vi "Host Train PID.vi"() -> ()   [LabVIEW 2018]
doc: "This example demonstrates the Traditional MeanShift algorithm to track an object in the image."
uses:
  <vilib>/userdefined/High Color/IMAQdx.ctl
  <vilib>/vision/driver/NI_Vision_Acquisition_Software.lvlib
panel:
  out "Control Signal":dbl(graph)
  out "DECODED MESSAGE":string
  in  "?":T1="cam1"
  in  "Run":bool
  out "Theta":cluster{"Double":dbl, dbl}(graph)
  in  "Stop":bool
  out "Image":T2(plugin-control)
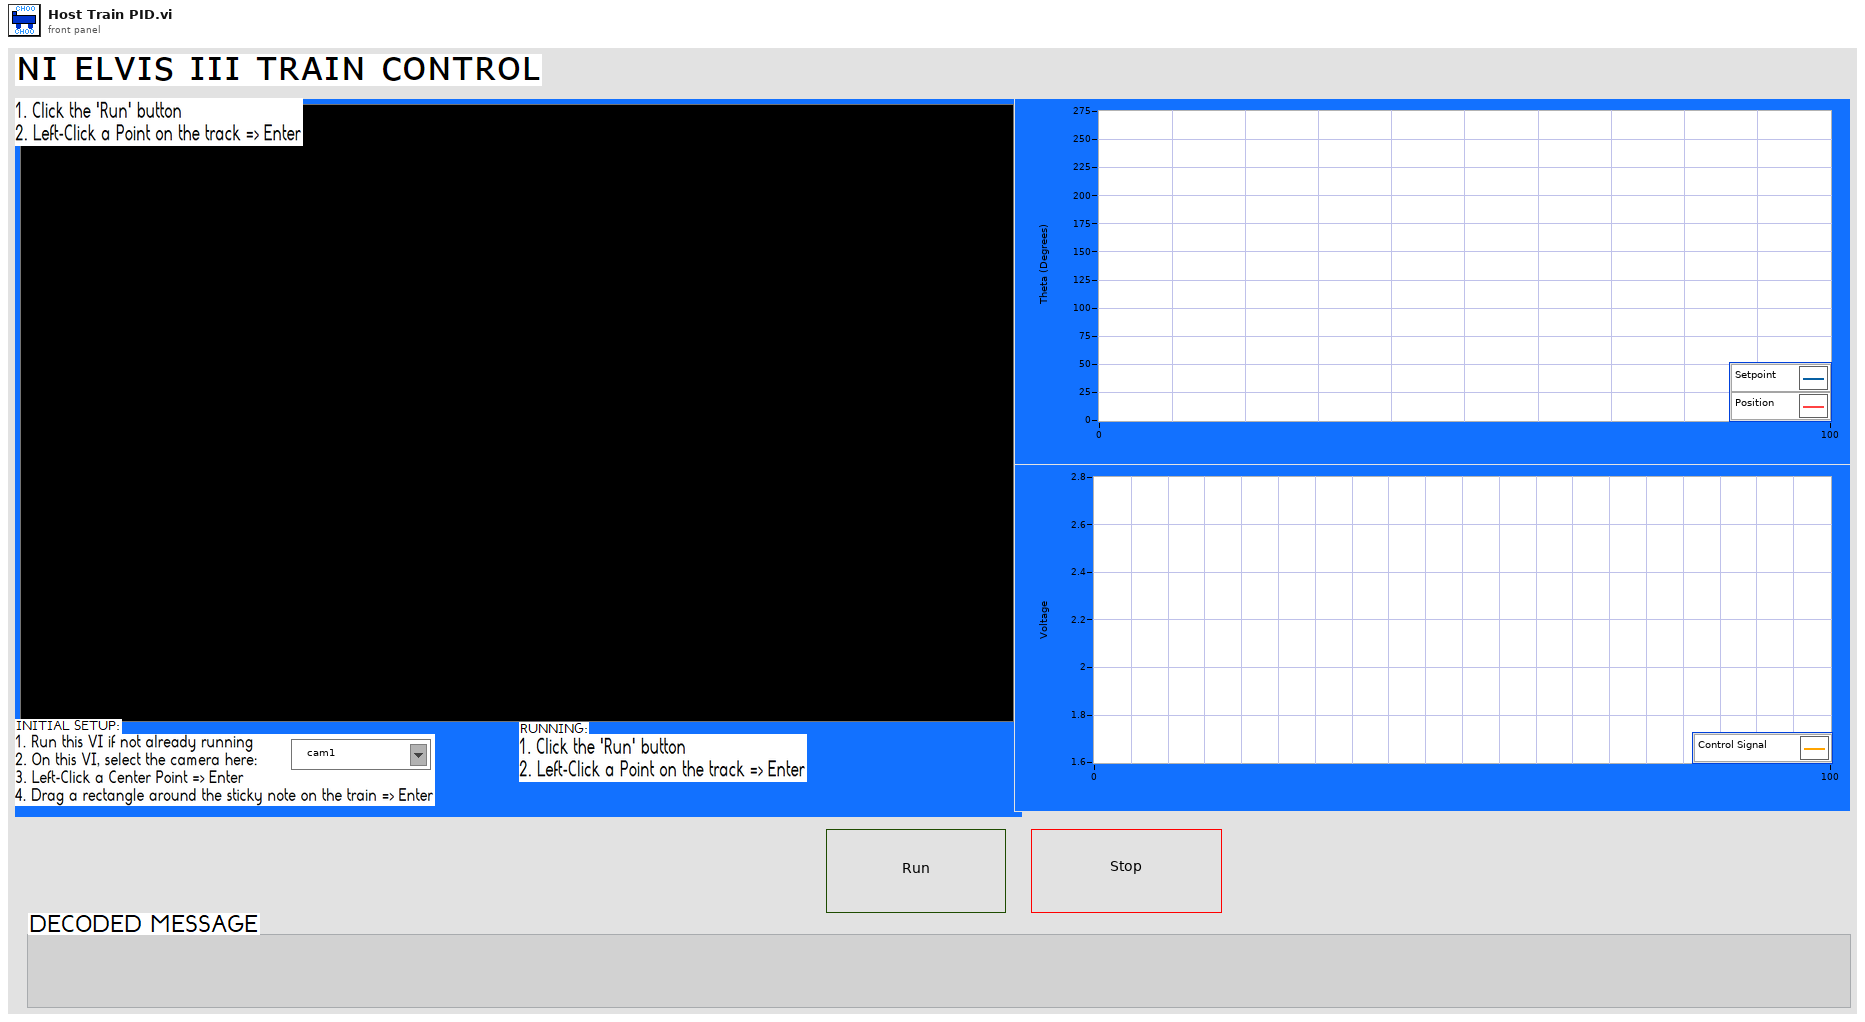
[diagram p1: front panel]
types:
  T1 = typedef "IMAQdx.ctl" = refnum<k21>
  T2 = typedef "IMAQ Image.ctl" = refnum<image>
  T3 = typedef "LVRectTypeDef.ctl" = cluster{"Left":i16, "Top":i16, "Right":i16, "Bottom":i16}
  T4 = typedef "IMAQ Object Tracking Session.ctl" = refnum<k20>
  T5 = typedef "IMAQ Point" = cluster{"X":sgl, "Y":sgl}
  T6 = cluster{"Label":string, "Score":i32, "Angle":dbl, "Location":cluster{"X":dbl, "Y":dbl}, "Bounding Box":cluster{"X":dbl, "Y":dbl}[], "Object Found?":bool}[]
  T7 = cluster{"Label":string, "Score":i32, "Angle":dbl, "Location":cluster{"X":dbl, "Y":dbl}, "Bounding Box":cluster{"X":dbl, "Y":dbl}[], "Object Found?":bool}
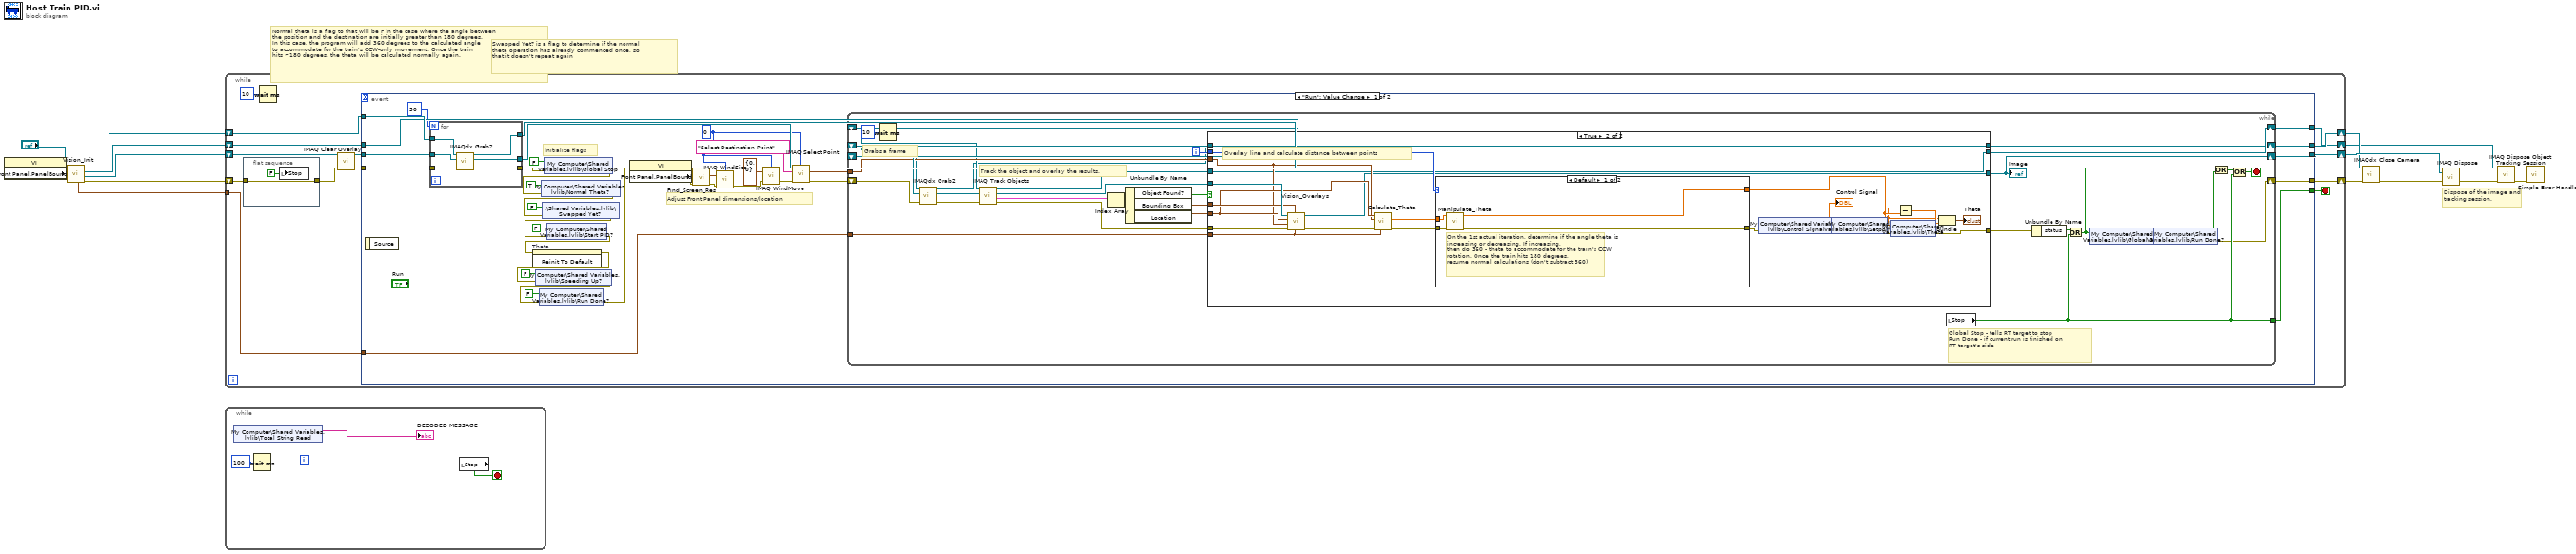
[diagram p0: block diagram]
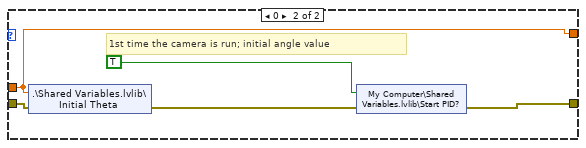
[diagram p3: hidden frame]
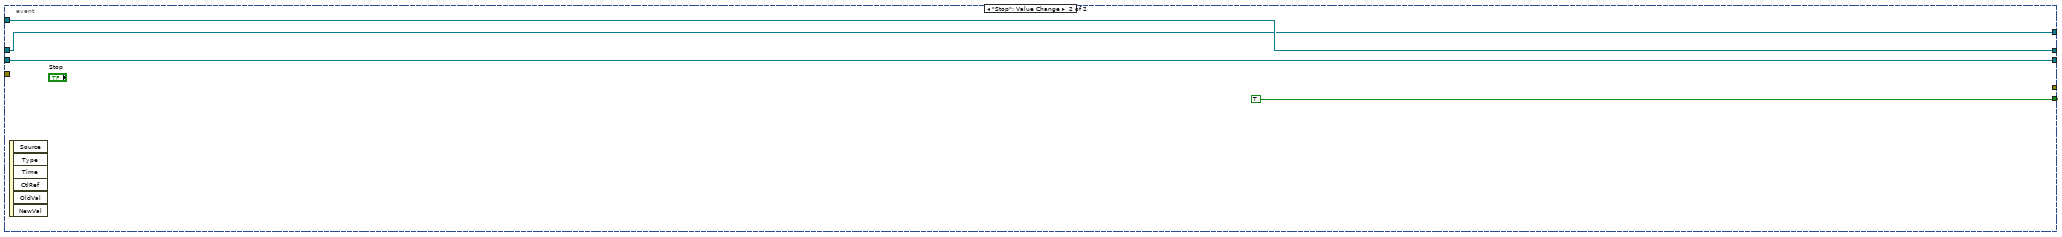
[diagram p4: hidden frame]
diagram:
  # "Swapped Yet? is a flag to determine if the normal\ntheta operation has already commenced once, so \nthat it doesn't repeat again"
  # "Normal theta is a flag to that will be F in the case where the angle between\nthe position and the destination are initially greater than 180 degrees. \nIn this case, the program will add 360 degrees to the calculated angle \nto accommodate for the train's CCW-only movement. Once the train\nhits ~180 degrees, the theta will be calculated normally again."
  # "Dispose of the image and tracking session."
  n1 = property class="VI"() -> ("Front Panel.PanelBounds"=w4:T3)  [unwired: 2 in, 2 out]
  n2 = call "Vision_Init.vi"("Front Panel.WinBounds"=w4, "Refnum in"="?") -> ("error out"=w9:errorcluster, "Image (duplicate)"=w10:T2, "Object Tracking Session Out"=w8:T4, "Refnum out"=w12:T1, "Center Point"=w7:T5)  [unwired: 5 in]
  n3 = while {
    tunnel: w7 -> [w26]
    shift-right: [w22] -> w5
    shift-left: w8 -> [w23]
    shift-right: [w28] -> w6
    shift-left: w12 -> [w24]
    shift-right: [w21] -> w11
    shift-left: w10 -> [w15]
    shift-right: [w27] -> w2
    shift-left: w9 -> [w20]
    stop <- w25 stop-if-true
    n4 = flat-sequence {
      tunnel: w20 -> [w29]
      tunnel: [w29] -> w17
      frame #0 {
        n5 = local write "Stop"(FALSE ("Stop")) -> ()
      }
    }
    n6 = Wait (ms)(milliseconds to wait=u32 10) -> ()  [unwired: 1 out]
    n7 = call "IMAQ Clear Overlay"("error in (no error)"=w17, "Image"=w15) -> ("error out"=w16:errorcluster, "Image Out"=w18:T2)  [unwired: 8 in]
    n8 = event shown="[0] \"Run\": Value Change" {
      selector: _ -> [_ _]
      dyn-events: _ -> [_ _]
      timeout: _ -> [_ _]
      tunnel: w23 -> [w56 w143]
      tunnel: [w69 w144] -> w28
      tunnel: [w32 _] -> w27
      tunnel: [w68 w142] -> w21
      tunnel: w18 -> [w57 w142]
      tunnel: w26 -> [w67 _]
      tunnel: [w66 TRUE ("Stop")] -> w25
      tunnel: w24 -> [w61 w144]
      tunnel: [w62 w143] -> w22
      tunnel: w16 -> [w44 _]
      event "Run": Value Change {
        w38 = 0 ("Window Number")
        # "Adjust Front Panel dimensions/location"
        # "Initialize flags"
        n9 = event-data() -> ()  [unwired: 1 in, 1 out]
        n10 = for {
          N: 50 -> [_]
          tunnel: w61 -> [w75]
          tunnel: [w74] -> w50
          tunnel: [w73] -> w59
          tunnel: [w72] -> w60
          tunnel: w57 -> [w71]
          tunnel: w44 -> [w70]
          n11 = call <vilib>:"IMAQdx Grab2.vi"("error in"=w70, "Image In"=w71, "Session In"=w75) -> ("error out"=w74:errorcluster, "Image Out"=w73:T2, "Session Out"=w72:T1)  [unwired: 5 in, 1 out]
        }
        n12 = shared-variable "My Computer\\Shared Variables.lvlib\\Global Stop"(FALSE ("Global Stop"), error in=w50) -> (error out=w49:errorcluster)
        n13 = shared-variable "My Computer\\Shared Variables.lvlib\\Normal Theta?"(TRUE ("Add 360?"), error in=w49) -> (error out=w48:errorcluster)
        n14 = shared-variable ".\\Shared Variables.lvlib\\Swapped Yet?"(FALSE ("Swapped Yet?"), error in=w48) -> (error out=w46:errorcluster)
        n15 = shared-variable "My Computer\\Shared Variables.lvlib\\Start PID?"(FALSE ("Start PID?"), error in=w46) -> (error out=w45:errorcluster)
        n16 = invoke on="Theta" class="WFChart (strict)" method="Reinit To Default"(error in=w45) -> (error out=w31:errorcluster)  [unwired: 2 in, 2 out]
        n17 = shared-variable "My Computer\\Shared Variables.lvlib\\Speeding Up?"(FALSE ("Speeding Up?"), error in=w31) -> (error out=w34:errorcluster)
        n18 = shared-variable "My Computer\\Shared Variables.lvlib\\Run Done?"(FALSE ("Run Done?"), error in=w34) -> (error out=w37:errorcluster)
        n19 = property class="VI"(error in=w37) -> (error out=w36:errorcluster, "Front Panel.PanelBounds"=w35:T3)  [unwired: 1 in, 1 out]
        n20 = call "Find_Screen_Res.vi"("error in (no error)"=w36, "Front Panel.WinBounds"=w35) -> ("error out"=w43:errorcluster, "Width & Height"=w42:cluster{"Width":i32, "Height":i32})  [unwired: 8 in]
        n21 = call "IMAQ WindSize"("error in (no error)"=w43, "Width & Height"=w42, "Window Number"=w38) -> ("error out"=w41:errorcluster)  [unwired: 3 in, 2 out]
        n22 = call "IMAQ WindMove"("Window Number (0...15)"=w38, "Coordinates (screen)"=cluster{"X Position":i32, "Y Position":i32} {"X Position"=0, "Y Position"=0}, "error in (no error)"=w41) -> ("error out"=w40:errorcluster)  [unwired: 2 in, 1 out]
        n23 = call "IMAQ Select Point"("Window Number (0...15)"=w38, "error in (no error)"=w40, "Prompt"="Select Destination Point", "Image In"=w59) -> ("error out"=w58:errorcluster, "Point"=w64:T5, "Image Out (duplicate)"=w63:T2)  [unwired: 4 in, 1 out]
        n24 = while {
          shift-right: [w76] -> w32
          shift-left: w58 -> [w106]
          shift-right: [w83] -> w69
          shift-left: w60 -> [w90]
          tunnel: w64 -> [w102]
          shift-right: [w82] -> w68
          shift-left: w63 -> [w103]
          tunnel: w67 -> [w101]
          tunnel: [w80] -> w66
          shift-right: [w85] -> w62
          shift-left: w56 -> [w89]
          i -> [w105]
          stop <- w99 stop-if-true
          # "Global Stop - tells RT target to stop\nRun Done - if current run is finished on\nRT target's side"
          # "Track the object and overlay the results."
          # "Grabs a frame"
          n25 = Wait (ms)(milliseconds to wait=u32 10) -> ()  [unwired: 1 out]
          n26 = call <vilib>:"IMAQdx Grab2.vi"("error in"=w106, "Image In"=w103, "Session In"=w90) -> ("error out"=w91:errorcluster, "Image Out"=w81:T2, "Session Out"=w84:T1)  [unwired: 5 in, 1 out]
          n27 = call "IMAQ Track Objects"("error in (no error)"=w91, "Image"=w81, "Object Tracking Session In"=w89) -> ("error out"=w95:errorcluster, "Objects (pixel)"=w98:T6, "Image (duplicate)"=w97:T2, "Object Tracking Session Out"=w86:T4)  [unwired: 1 in, 4 out]
          n28 = Index Array(array=w98) -> (element=w94:T7)  [unwired: 1 in]
          n29 = Unbundle By Name(w94) -> ("Object Found?"=w93:bool, "Bounding Box"=w96:cluster{"X":dbl, "Y":dbl}[], "Location"=w92:cluster{"X":dbl, "Y":dbl})
          n30 = case shown="True" w93 {
            tunnel: w97 -> [w109 w132]
            tunnel: [w109 w114] -> w82
            tunnel: w96 -> [_ w130]
            tunnel: w95 -> [w110 w131]
            tunnel: [w110 w117] -> w77
            tunnel: w92 -> [_ w129]
            tunnel: w102 -> [_ w128]
            tunnel: w101 -> [_ w126]
            tunnel: w105 -> [_ w125]
            tunnel: w86 -> [w107 w120]
            tunnel: [w107 w120] -> w85
            tunnel: w84 -> [w108 w119]
            tunnel: [w108 w119] -> w83
            frame False {
            }
            frame True {
              # "Overlay line and calculate distance between points"
              n31 = call "Vision_Overlays.vi"("Center"=w126, "Bounding Box"=w130, "error in (no error)"=w131, "Destination"=w128, "Position"=w129, "Image in"=w132) -> ("error out"=w127:errorcluster, "Image out"=w114:T2)  [unwired: 4 in]
              n32 = call "Calculate_Theta.vi"("Center"=w126, "error in"=w127, "Destination"=w128, "Position"=w129) -> ("error out"=w124:errorcluster, "Theta"=w123:dbl)  [unwired: 6 in]
              n33 = case shown="Default" w125 {
                tunnel: w123 -> [w136 w140]
                tunnel: w124 -> [w133 w141]
                tunnel: [w134 w137] -> w113
                tunnel: [w135 w140] -> w116
                frame Default {
                  # "On the 1st actual iteration, determine if the angle theta is increasing or decreasing. If increasing, \nthen do 360 - theta to accommodate for the train's CCW rotation. Once the train hits 180 degrees,\nresume normal calculations (don't subtract 360)"
                  n34 = call "Manipulate_Theta.vi"("error in (no error)"=w133, "Theta in"=w136) -> ("error out"=w134:errorcluster, "Theta out"=w135:dbl)  [unwired: 7 in, 1 out]
                }
                frame 0 {
                  # "1st time the camera is run; initial angle value"
                  n35 = shared-variable ".\\Shared Variables.lvlib\\Initial Theta"(w140, error in=w141) -> (error out=w138:errorcluster)
                  n36 = shared-variable "My Computer\\Shared Variables.lvlib\\Start PID?"(TRUE ("Start PID?"), error in=w138) -> (error out=w137:errorcluster)
                }
              }
              n37 = shared-variable "My Computer\\Shared Variables.lvlib\\Control Signal"(error in=w113) -> (→"Control Signal":dbl, error out=w112:errorcluster)
              n38 = shared-variable "My Computer\\Shared Variables.lvlib\\Setpoint"(error in=w112) -> (w115:dbl, error out=w118:errorcluster)
              n39 = shared-variable "My Computer\\Shared Variables.lvlib\\Theta"(w116, error in=w118) -> (error out=w117:errorcluster)
              n40 = Subtract(x=w115, y=w116) -> (x-y=w121:dbl)
              n41 = Bundle("Double"=w115, w121) -> (→"Theta":cluster{"Double":dbl, dbl})  [unwired: 1 in]
            }
          }
          "Image" <- w82
          n42 = local read "Stop"() -> (w80:bool)
          n43 = Unbundle By Name(w77) -> ("status"=w100:bool)
          n44 = Or(x=w100, y=w80) -> (x .or. y?=w88:bool)
          n45 = shared-variable "My Computer\\Shared Variables.lvlib\\Global Stop"(w88) -> (error out=w78:errorcluster)  [unwired: 1 in]
          n46 = shared-variable "My Computer\\Shared Variables.lvlib\\Run Done?"(error in=w78) -> (w79:bool, error out=w76:errorcluster)
          n47 = Or(x=w88, y=w79) -> (x .or. y?=w87:bool)
          n48 = Or(x=w87, y=w80) -> (x .or. y?=w99:bool)
        }
      }
      event "Stop": Value Change {
        n49 = event-data() -> ()  [unwired: 1 in, 6 out]
      }
    }
  }
  n50 = while {
    stop <- w147 stop-if-true
    n51 = shared-variable "My Computer\\Shared Variables.lvlib\\Total String Read"() -> (→"DECODED MESSAGE":string)  [unwired: 1 in, 1 out]
    n52 = Wait (ms)(milliseconds to wait=u32 100) -> ()  [unwired: 1 out]
    n53 = local read "Stop"() -> (w147:bool)
  }
  n54 = call <vilib>:"IMAQdx Close Camera.vi"("error in"=w2, "Session In"=w6) -> ("error out"=w3:errorcluster)  [unwired: 9 in]
  n55 = call "IMAQ Dispose"("Image"=w11, "error in (no error)"=w3) -> ("error out"=w14:errorcluster)  [unwired: 1 in, 3 out]
  n56 = call "IMAQ Dispose Object Tracking Session"("error in (no error)"=w14, "Object Tracking Session"=w5) -> ("error out"=w13:errorcluster)  [unwired: 9 out]
  n57 = call <vilib>:"Simple Error Handler.vi"("error in (no error)"=w13) -> ()  [unwired: 1 in, 8 out]
